vi "Transmit.vi"(8 "error in (no error)":errorcluster, 10 "Transfer Group in":refnum<class "Transfer Group.lvclass">, 11 "Transceiver in":refnum<class "Transceiver.lvclass">) -> (0 "error out":errorcluster, 2 "Transfer Group out":refnum<class "Transfer Group.lvclass">, 3 "Transceiver out":refnum<class "Transceiver.lvclass">)   [LabVIEW 2017, in "Data Sharing Framework Core.lvlib" / "Data Sharing Framework Engine.lvlib" / "Transceiver.lvclass"]
uses:
  Transceiver.lvclass
  Transfer Group/Transfer Group.lvclass
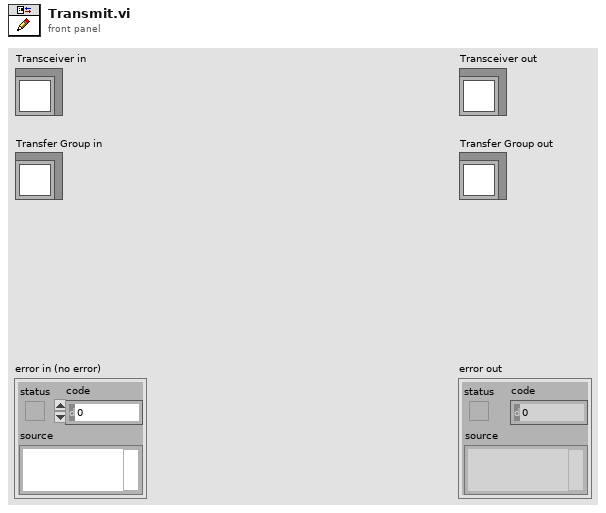
[diagram p1: front panel]
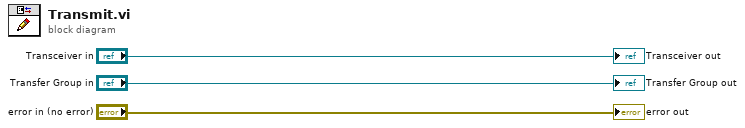
[diagram p0: block diagram]
diagram:
  "error out" <- "error in (no error)"
  "Transceiver out" <- "Transceiver in"
  "Transfer Group out" <- "Transfer Group in"
